vi "Get Bit (U32).vi"(10 "Bit":u8, 11 "Number":u32 format="%.0x") -> (2 "Value":bool=TRUE, 3 "Number Out":u32 format="%.0x")   [LabVIEW 2019, in "Bits.lvlib"]
doc: "Returns the bit value of the bit in the passed in number."
uses:
  Bits.lvlib
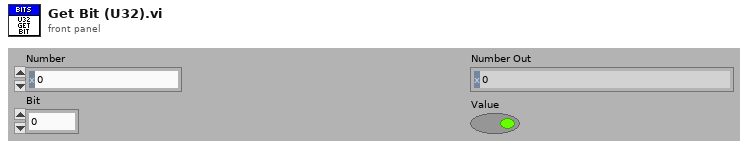
[diagram p1: front panel]
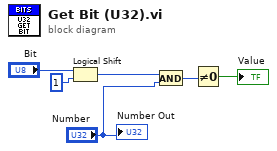
[diagram p0: block diagram]
diagram:
  n1 = Logical Shift(y="Bit", x=u32 1) -> (x << y=w4:u32)
  n2 = And(x=w4, y="Number") -> (x .and. y?=w2:u32)
  n3 = Not Equal To 0?(x=w2) -> (x != 0?=→"Value":bool)
  "Number Out" <- "Number"
